vi "Build Array (JSON).vi"(8 "error in (no error)":errorcluster, 10 "JSON Datatype":refnum<class "JSON Datatype.lvclass">=refnum, 11 "JSON Array in":refnum<class "JSON Array.lvclass">=refnum) -> (0 "error out":errorcluster, 3 "JSON Array out":refnum<class "JSON Array.lvclass">)   [LabVIEW 2017]
uses:
  JSON Datatype/JSON Datatype.lvclass
  JSON Array.lvclass
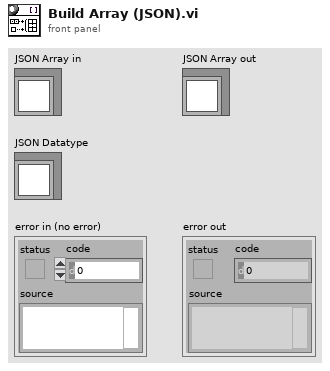
[diagram p1: front panel]
types:
  T1 = typedef "JSON Types.ctl" = enum16{"String", "Numeric", "Boolean", "NULL", "Object", "1D Array", "1D String", "1D Numeric", "1D Boolean"}
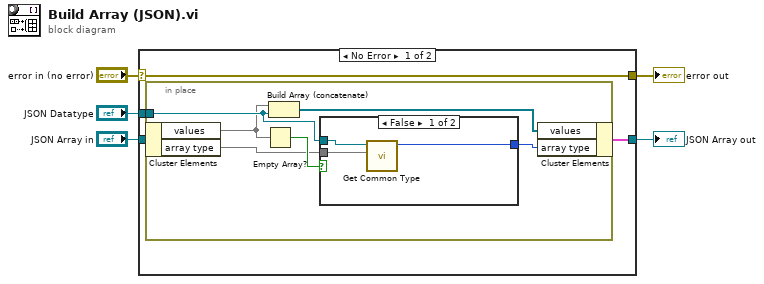
[diagram p0: block diagram]
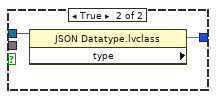
[diagram p2: hidden frame]
diagram:
  n1 = case shown="No Error" "error in (no error)" {
    selector: "error in (no error)" -> [w9 w22]
    tunnel: [w9 w22] -> w4
    tunnel: [w6 w21] -> w2
    tunnel: "JSON Array in" -> [w8 w21]
    tunnel: "JSON Datatype" -> [w7 _]
    frame No Error {
      n2 = in-place {
        in-place-border: w7 -> [w13]
        n3 = in-place-cluster #1(w8) -> ("values"=w10, "array type"=w12)
        n4 = Empty Array?(array=w10) -> (empty?=w14:bool)
        n5 = Build Array (concatenate)(w10, w13) -> (w15:refnum<class "JSON Datatype.lvclass">[])
        n6 = case shown="False" w14 {
          tunnel: w13 -> [w18 w20]
          tunnel: w12 -> [w17 _]
          tunnel: [w16 w19] -> w11
          frame False {
            n7 = call "Get Common Type.vi"("array type"=w17, "JSON Datatype in"=w18) -> ("type"=w16:T1)  [unwired: 9 in]
          }
          frame True {
            n8 = property class="JSON Datatype.lvclass"(reference=w20) -> ("type"=w19)  [unwired: 1 in, 2 out]
          }
        }
        n9 = in-place-cluster #1("values"=w15, "array type"=w11) -> (w6:cluster{})
      }
    }
    frame Error {
    }
  }
  "error out" <- w4
  "JSON Array out" <- w2
